vi "From.vi"(1 "String":string) -> (0 "String":refnum<class "String.lvclass">)   [LabVIEW 2018, in "Toolkit.lvlib" / "Readers.lvlib" / "String.lvclass"]
uses:
  String.lvclass
  String.lvclass/String.ctl
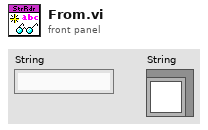
[diagram p1: front panel]
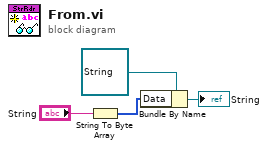
[diagram p0: block diagram]
diagram:
  n1 = String To Byte Array(string="String") -> (unsigned byte array=w2:u8[])
  n2 = Bundle By Name(cluster=refnum<class "String.lvclass"> refnum ("Mustache.lvlib:Readers.lvlib:String.lvclass"), "Data"=w2) -> (→"String":refnum<class "String.lvclass">)
